vi "Test Worker Waiting After Completing Job.vi"(8 "error in (no error)":errorcluster, 11 "Barista Test in":refnum<class "Barista Test.lvclass">=refnum) -> (0 "error out":errorcluster, 3 "Barista Test out":refnum<class "Barista Test.lvclass">)   [LabVIEW 2020, in "Barista Test.lvclass"]
uses:
  Barista Test.lvclass
  Worker Test/Worker Test.lvclass
  <vilib>/Astemes/Triarc Framework/Process/Process.lvclass
  <vilib>/Astemes/LUnit/Test Case.lvclass
  Processes/People/Workers/Worker/Worker.lvclass
  Test Doubles/Stub Job Handler/Stub Job Handler.lvclass
  Support/Order Item/Order Item.lvclass
  Support/Beverages/Beverage/Beverage.lvclass
  C:/git/astemes-triarc-examples/source/Coffee Shop/Processes/People/Person/Person.lvclass
  C:/Program Files (x86)/National Instruments/LabVIEW 2020/vi.lib/Astemes/Triarc Framework/View/View.lvclass
  C:/Program Files (x86)/National Instruments/LabVIEW 2020/vi.lib/Astemes/Triarc Framework/Process/Process.lvclass
  C:/Program Files (x86)/National Instruments/LabVIEW 2020/vi.lib/Astemes/Triarc Framework/Base/Base.lvclass
  C:/Program Files (x86)/National Instruments/LabVIEW 2020/vi.lib/Astemes/Triarc Framework/Error Handler Interface/Error Handler Interface.lvclass
  C:/Program Files (x86)/National Instruments/LabVIEW 2020/vi.lib/Astemes/Triarc Framework/Logging/Logging.lvclass
  C:/git/astemes-triarc-examples/source/Coffee Shop/Processes/People/Workers/Worker/Worker.lvclass
  C:/git/astemes-triarc-examples/source/Coffee Shop/Processes/People/Process Job/Job Handler.lvclass
  <vilib>/Astemes/Triarc Framework/Support/Broadcast Event Dequeuers.lvlib
  C:/Program Files (x86)/National Instruments/LabVIEW 2020/vi.lib/Astemes/LUnit/Test Case.lvclass
  C:/Program Files (x86)/National Instruments/LabVIEW 2020/vi.lib/Astemes/LUnit/LUnit Runnable.lvclass
  C:/git/astemes-triarc-examples/source/Coffee Shop/Tests/Test Doubles/Stub Job Handler/Stub Job Handler.lvclass
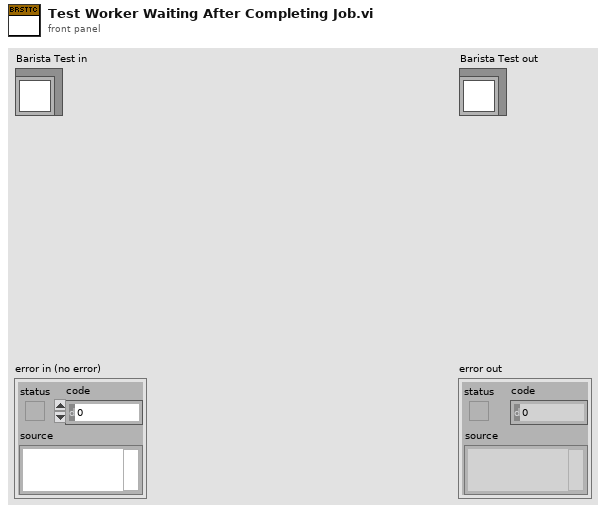
[diagram p1: front panel]
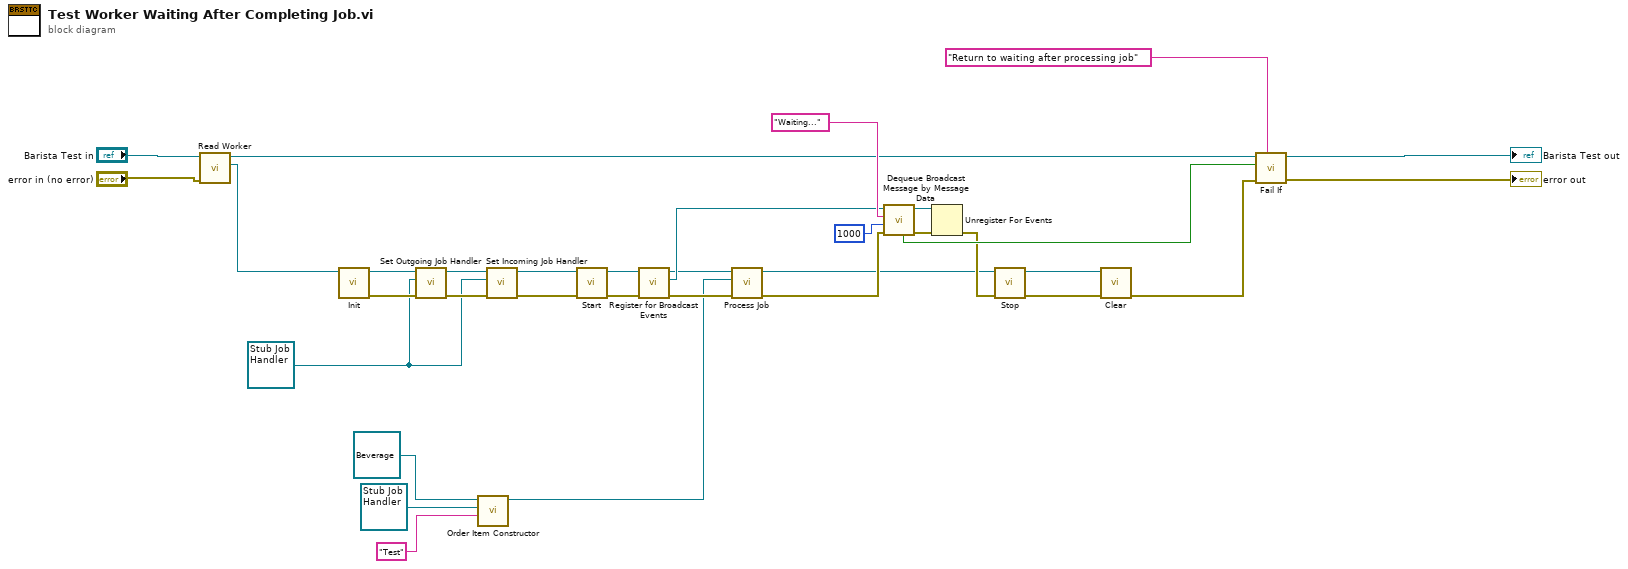
[diagram p0: block diagram]
diagram:
  w1 = refnum<class "Stub Job Handler.lvclass"> refnum ("Stub Job Processor.lvclass")
  n1 = call "Read Worker.vi"("error in (no error)"="error in (no error)", "Worker Test in"="Barista Test in") -> ("Worker"=w7:refnum<class "Worker.lvclass">, "Worker Test out"=w6:refnum<class "Worker Test.lvclass">)  [unwired: 7 in, 1 out]
  n2 = call-dynamic "Init.vi"("View In"=w7) -> ("error out"=w26:errorcluster, "View Out"=w25:refnum<class "Worker.lvclass">)  [unwired: 9 in]
  n3 = call "Set Outgoing Job Handler.vi"("error in (no error)"=w26, "Work Dispatcher"=w1, "Worker In"=w25) -> ("error out"=w30:errorcluster, "Worker Out"=w27:refnum<class "Worker.lvclass">)  [unwired: 7 in]
  n4 = call "Order Item Constructor.vi"("Cust Name"="Test", "Pick Up Order Handler"=refnum<class "Stub Job Handler.lvclass"> refnum ("Stub Job Handler.lvclass"), "Beverage"=refnum<class "Beverage.lvclass"> refnum) -> ("Order Item"=w2:refnum<class "Order Item.lvclass">)  [unwired: 7 in, 1 out]
  n5 = call "Set Incoming Job Handler.vi"("error in (no error)"=w30, "Job Handler"=w1, "Worker In"=w27) -> ("error out"=w29:errorcluster, "Worker Out"=w28:refnum<class "Worker.lvclass">)  [unwired: 7 in]
  n6 = call <vilib>:"Start.vi"("error in (no error)"=w29, "Process In"=w28) -> ("error out"=w10:errorcluster, "Process Out"=w14:refnum<class "Worker.lvclass">)  [unwired: 7 in, 1 out]
  n7 = call <vilib>:"Register for Broadcast Events.vi"("error in (no error)"=w10, "Process In"=w14) -> ("error out"=w13:errorcluster, "Event Registration Refnum Out"=w18:refnum<event-registration>, "Process Out"=w15:refnum<class "Worker.lvclass">)  [unwired: 7 in]
  n8 = call-dynamic "Process Job.vi"("error in (no error)"=w13, "Job"=w2, "Worker In"=w15) -> ("error out"=w17:errorcluster, "Worker Out"=w16:refnum<class "Worker.lvclass">)  [unwired: 7 in]
  n9 = call <vilib>:"Dequeue Broadcast Message by Message Data.vi"("error in (no error)"=w17, "Timeout (-1)"=1000, "Message Data"="Waiting...", "Event Registration Refnum"=w18) -> ("error out"=w21:errorcluster, "Event Registration Refnum Out"=w23:refnum<event-registration>, "Timed Out?"=w24:bool)  [unwired: 3 in, 2 out]
  n10 = Unregister For Events(event registration refnum=w23, error in=w21) -> (error out=w22:errorcluster)
  n11 = call <vilib>:"Stop.vi"("error in (no error)"=w22, "Process In"=w16) -> ("error out"=w9:errorcluster, "Process Out"=w8:refnum<class "Worker.lvclass">)  [unwired: 7 in, 1 out]
  n12 = call-dynamic "Clear.vi"("error in (no error)"=w9, "View In"=w8) -> ("error out"=w11:errorcluster)  [unwired: 9 in]
  n13 = call <vilib>:"Fail If.vi"("Description"="Return to waiting after processing job", "error in (no error)"=w11, "Fail?"=w24, "LUnit Test Case In"=w6) -> ("error out"=→"error out":errorcluster, "LUnit Test Case Out"=→"Barista Test out":refnum<class "Test Case.lvclass">)  [unwired: 6 in]
